vi "Tosca-Stop DI.vi"(0 "Refnum in":refnum<k21>, 11 "error in (no error)":errorcluster) -> ()   [LabVIEW 2020]
uses:
  epl-vi-lib/PXI DAQ VIs/TDT VIs/TDT-Globals.vi
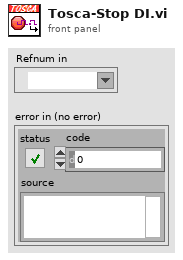
[diagram p1: front panel]
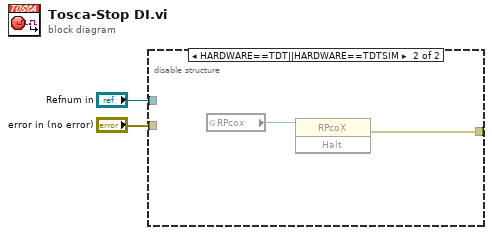
[diagram p0: block diagram]
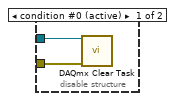
[diagram p2: hidden frame]
diagram:
  n1 = disable-structure shown="HARDWARE==TDT||HARDWARE==TDTSIM" {
    disable-tunnel: "Refnum in" -> [w4 _]
    disable-tunnel: "error in (no error)" -> [w3 _]
    disable-tunnel: [_ w5] -> _
    frame condition #0 (active) {
      n2 = call <vilib>:"DAQmx Clear Task.vi"("task in"=w4, "error in"=w3) -> ()  [unwired: 13 in, 1 out]
    }
    frame condition #1 {
      n3 = global read "TDT-Globals.vi" "RPcox"() -> (w6:refnum<k7>)
      n4 = invoke class="RPcoX" method="Halt"(reference=w6) -> (error out=w5:errorcluster)  [unwired: 2 in, 2 out]
    }
  }
